vi "Write TIFF Header.vi"(0 "File Path":path, 7 "Image Info":T2, 11 "Error":errorcluster) -> (4 "File Ref":refnum<file>, 8 "Byte Order":T1(ring), 15 "Error":errorcluster)   [LabVIEW 2016]
uses:
  IFD Entry.ctl
  TIF Write Image Information.ctl
panel:
  out "TIF Description":string
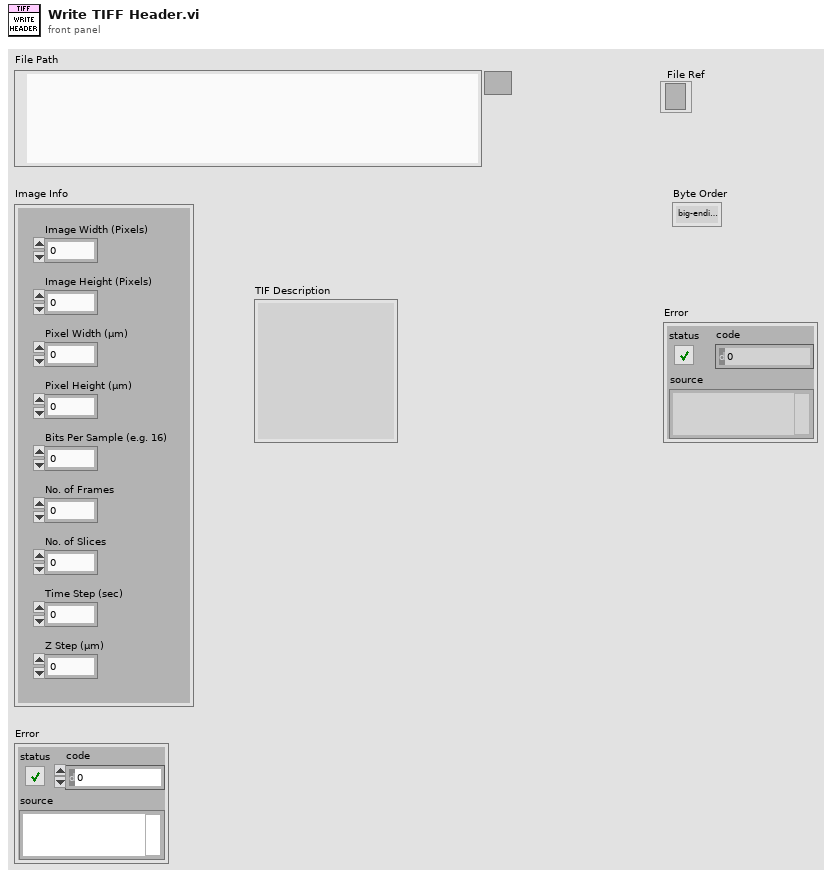
[diagram p1: front panel]
types:
  T1 = enum16{"big-endian, network order", "native, host order", "little-endian"}
  T2 = typedef "TIF Write Image Information.ctl" = cluster{"Image Width (Pixels)":u32, "Image Height (Pixels)":u32, "Pixel Width (µm)":dbl, "Pixel Height (µm)":dbl, "Bits Per Sample (e.g. 16)":u32, "No. of Frames":u32, "No. of Slices":u32, "Time Step (sec)":dbl, "Z Step (µm)":dbl}
  T3 = typedef "IFD Entry.ctl" = cluster{"TIF Tag (U16)":u16, "Data Type (U16)":u16, "Count (U32)":u32, "Value or Offset (U32)":u32, "Write Offset (I64)":i64}
  T4 = enum16{"open", "replace", "create", "open or create", "replace or create", "replace or create with confirmation"}
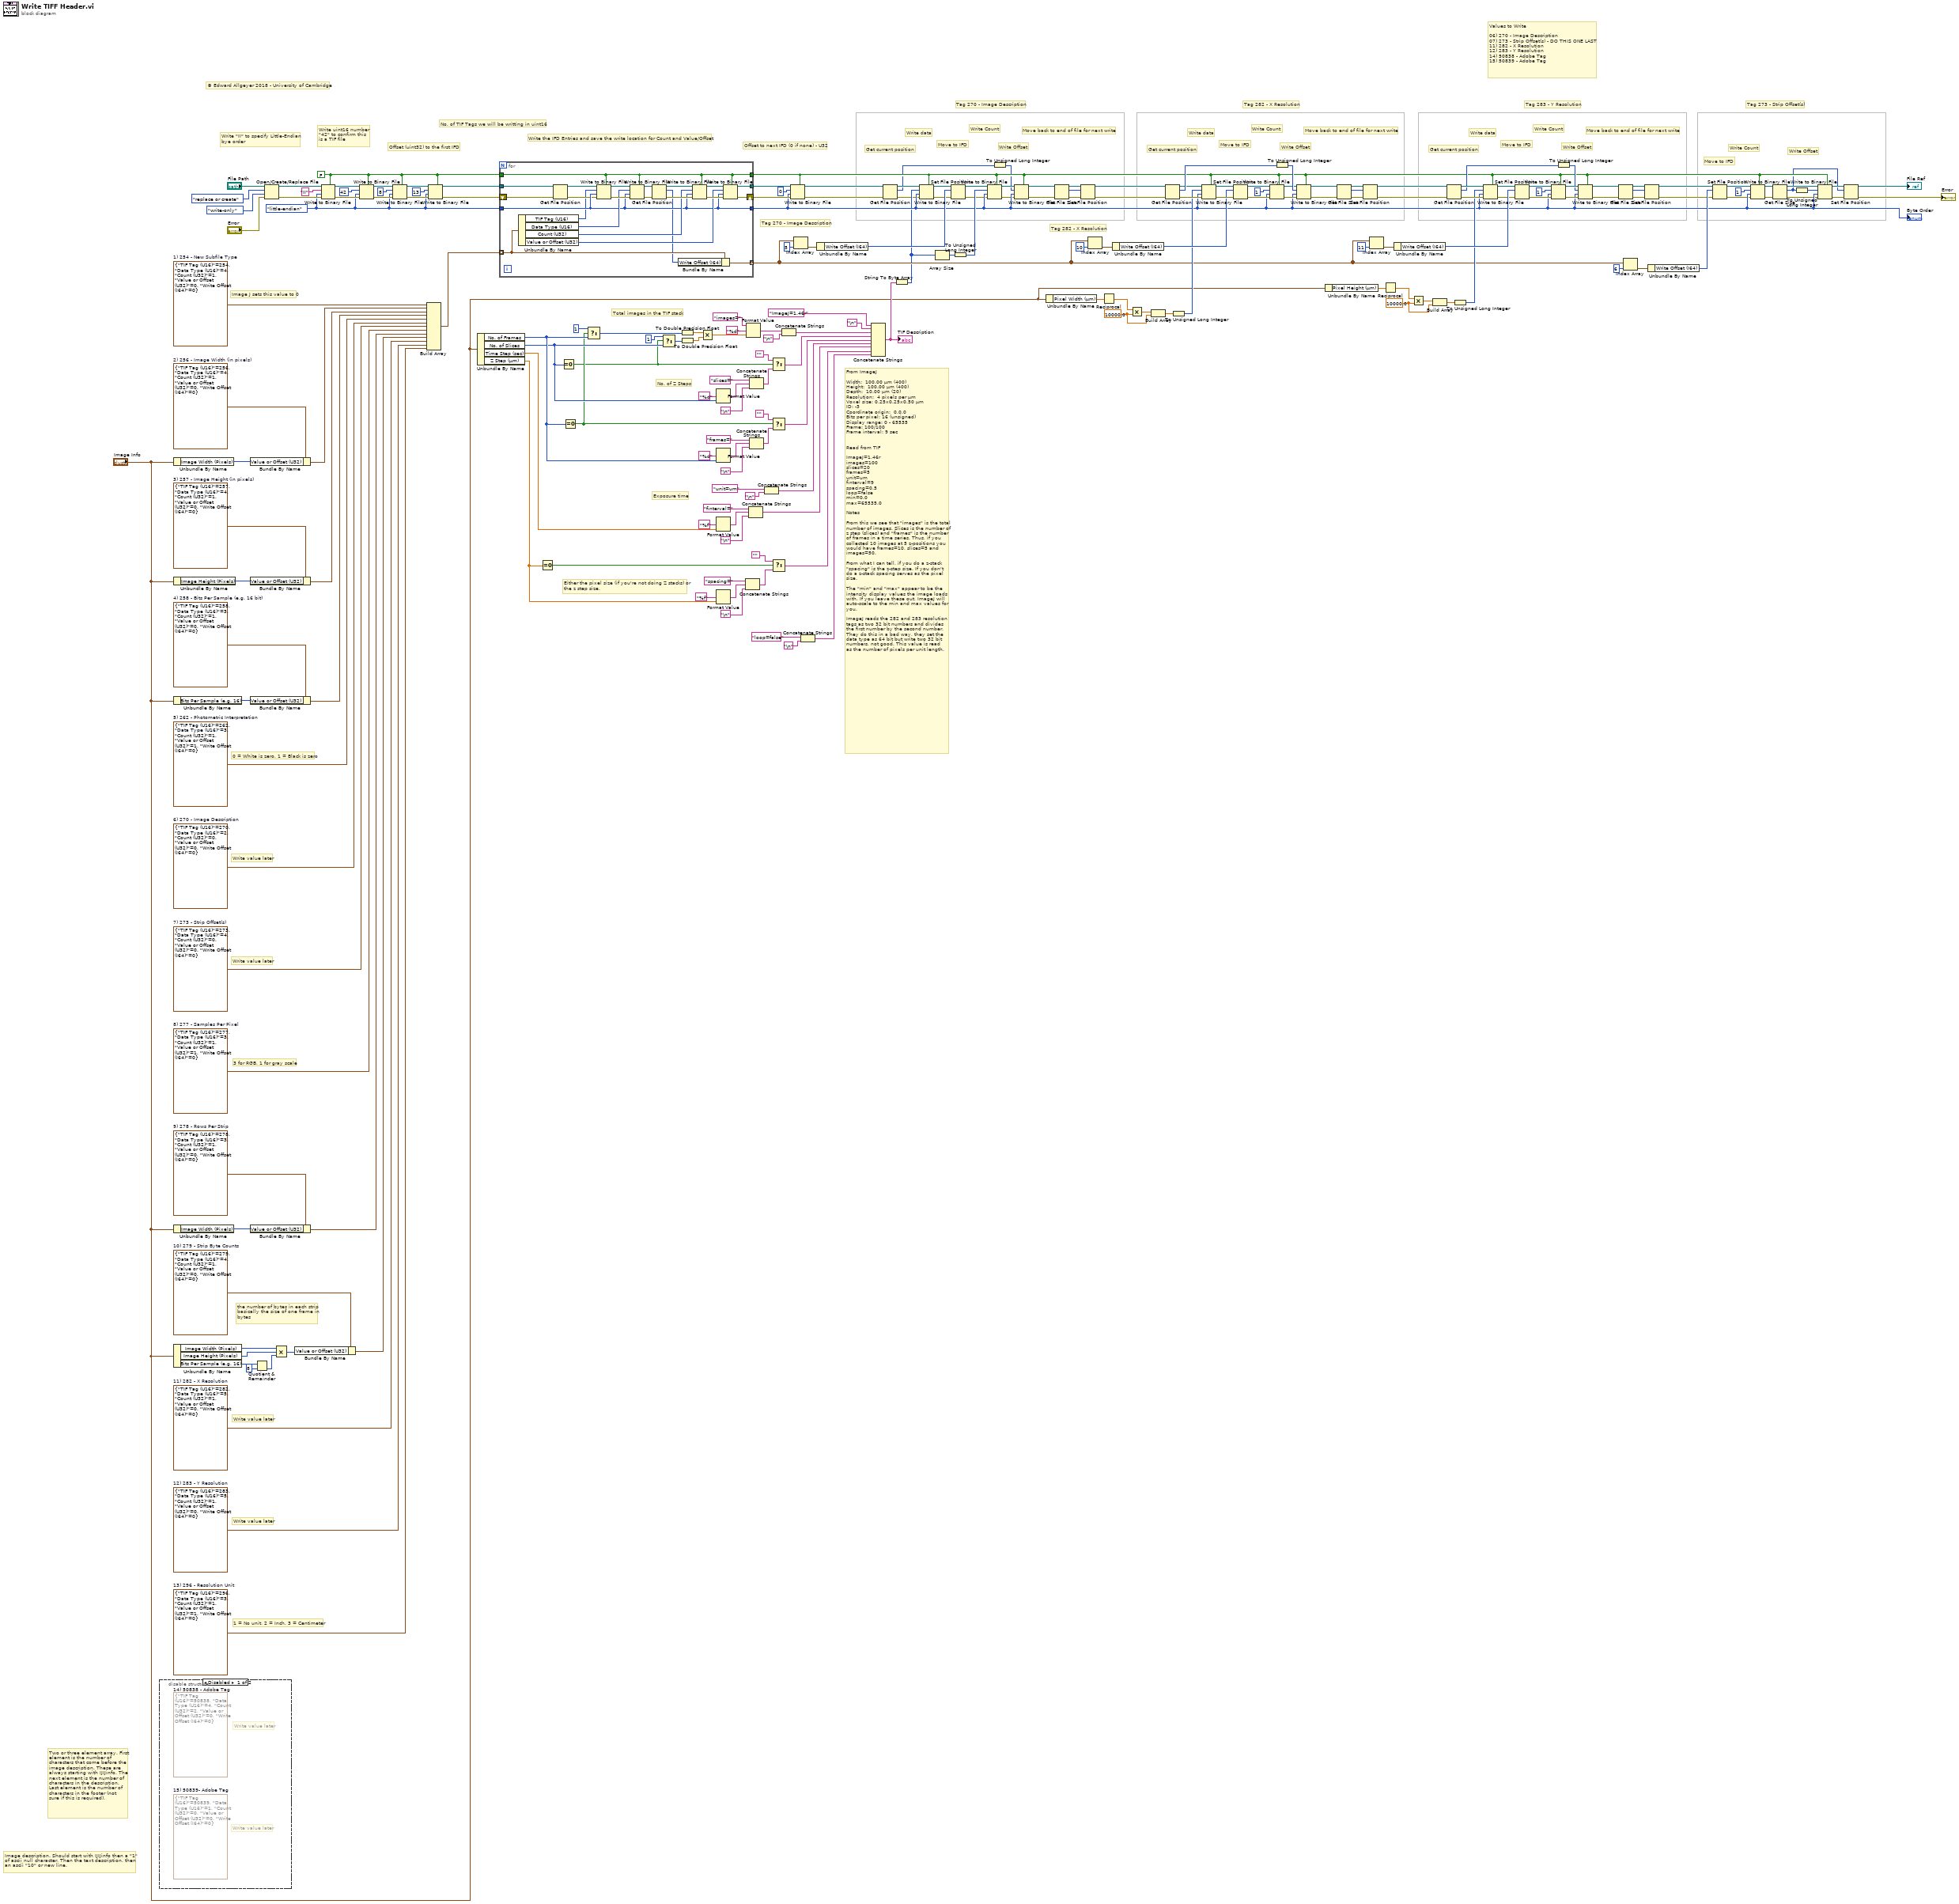
[diagram p0: block diagram]
diagram:
  w82 = 10000.0 ("y")
  w86 = 10000.0 ("y")
  w163 = T3 {"TIF Tag (U16)"=296, "Data Type (U16)"=3, "Count (U32)"=1, "Value or Offset (U32)"=1, "Write Offset (I64)"=0}  # 13) 296 - Resolution Unit
  w164 = T3 {"TIF Tag (U16)"=283, "Data Type (U16)"=5, "Count (U32)"=1, "Value or Offset (U32)"=0, "Write Offset (I64)"=0}  # 12) 283 - Y Resolution
  w165 = T3 {"TIF Tag (U16)"=282, "Data Type (U16)"=5, "Count (U32)"=1, "Value or Offset (U32)"=0, "Write Offset (I64)"=0}  # 11) 282 - X Resolution
  w168 = T3 {"TIF Tag (U16)"=279, "Data Type (U16)"=4, "Count (U32)"=1, "Value or Offset (U32)"=0, "Write Offset (I64)"=0}  # 10) 279 - Strip Byte Counts
  w176 = T3 {"TIF Tag (U16)"=278, "Data Type (U16)"=3, "Count (U32)"=1, "Value or Offset (U32)"=0, "Write Offset (I64)"=0}  # 9) 278 - Rows Per Strip
  w177 = T3 {"TIF Tag (U16)"=277, "Data Type (U16)"=3, "Count (U32)"=1, "Value or Offset (U32)"=1, "Write Offset (I64)"=0}  # 8) 277 - Samples Per Pixel
  w178 = T3 {"TIF Tag (U16)"=273, "Data Type (U16)"=4, "Count (U32)"=0, "Value or Offset (U32)"=0, "Write Offset (I64)"=0}  # 7) 273 - Strip Offset(s)
  w179 = T3 {"TIF Tag (U16)"=270, "Data Type (U16)"=2, "Count (U32)"=0, "Value or Offset (U32)"=0, "Write Offset (I64)"=0}  # 6) 270 - Image Description
  w180 = T3 {"TIF Tag (U16)"=262, "Data Type (U16)"=3, "Count (U32)"=1, "Value or Offset (U32)"=1, "Write Offset (I64)"=0}  # 5) 262 - Photometric Interpretation
  w183 = T3 {"TIF Tag (U16)"=258, "Data Type (U16)"=3, "Count (U32)"=1, "Value or Offset (U32)"=0, "Write Offset (I64)"=0}  # 4) 258 - Bits Per Sample (e.g. 16 bit)
  w186 = T3 {"TIF Tag (U16)"=257, "Data Type (U16)"=4, "Count (U32)"=1, "Value or Offset (U32)"=0, "Write Offset (I64)"=0}  # 3) 257 - Image Height (in pixels)
  w190 = T3 {"TIF Tag (U16)"=256, "Data Type (U16)"=4, "Count (U32)"=1, "Value or Offset (U32)"=0, "Write Offset (I64)"=0}  # 2) 256 - Image Width (in pixels)
  w188 = T3 {"TIF Tag (U16)"=254, "Data Type (U16)"=4, "Count (U32)"=1, "Value or Offset (U32)"=0, "Write Offset (I64)"=0}  # 1) 254 - New Subfile Type
  w158 = FALSE ("prepend array or string size? (T)")
  w159 = T1."little-endian" ("byte order (0:big-endian, network order)")
  # "© Edward Allgeyer 2018 - University of Cambridge"
  # "No. of Z Steps"
  # "Either the pixel size (if you're not doing Z stacks) or\nthe z step size."
  # "Total images in the TIF stack"
  # "Exposure time"
  # "Tag 270 - Image Description"
  # "Move back to end of file for next write"
  # "Move to IFD"
  # "Write data"
  # "Get current position"
  # "Write Offset"
  # "Write Count"
  # "Tag 273 - Strip Offset(s)"
  # "Move to IFD"
  # "Write Offset"
  # "Write Count"
  # "Tag 283 - Y Resolution"
  # "Move back to end of file for next write"
  # "Move to IFD"
  # "Write data"
  # "Get current position"
  # "Write Offset"
  # "Write Count"
  # "Tag 282 - X Resolution"
  # "Tag 282 - X Resolution"
  # "Move back to end of file for next write"
  # "Move to IFD"
  # "Write data"
  # "Get current position"
  # "Write Offset"
  # "Write Count"
  # "Offset to next IFD (0 if none) - U32"
  # "Tag 270 - Image Description"
  # "From ImageJ\n\nWidth:  100.00 µm (400)\nHeight:  100.00 µm (400)\nDepth:  10.00 µm (20)\nResolution:  4 pixels per µm\nVoxel size: 0.25x0.25x0.50 µm\nID: -3\nCoordinate origin:  0,0,0\nBits per pixel: 16 (unsigned)\nDisplay range: 0 - 65535\nFrame: 100/100\nFrame interval: 9 sec\n\n\nRead from TIF\n\nImageJ=1.46r\nimages=100\nslices=20\nframes=5\nunit=um\nfinterval=9\nspacing=0.5\nloop=false\nmin=0.0\nmax=65535.0\n\nNotes\n\nFrom this we see that \"images\" is the total\nnumber of images. Slices is the number of\nz step (slices) and \"frames\" is the number\nof frames in a time series. Thus, if you\ncollected 10 images at 5 z-positions you\nwould have frames=10, slices=5 and\nimages=50.\n\nFrom what I can tell, if you do a z-stack\n\"spacing\" is the z-step size. If you don't\ndo a z-stack spacing serves as the pixel\nsize.\n\nThe \"min\" and \"max\" appear to be the\nintensity display values the image loads\nwith. If you leave these out, ImageJ will\nauto-scale to the min and max values for\nyou.\n\nImageJ reads the 282 and 283 resolution\ntags as two 32 bit numbers and divides\nthe first number by the second number.\nThey do this in a bad way, they set the\ndata type as 64 bit but write two 32 bit\nnumbers, not good. This value is read\nas the number of pixels per unit length."
  # "Values to Write\n\n06) 270 - Image Description\n07) 273 - Strip Offset(s) - DO THIS ONE LAST\n11) 282 - X Resolution\n12) 283 - Y Resolution\n14) 50838 - Adobe Tag\n15) 50839 - Adobe Tag"
  # "Write the IFD Entries and save the write location for Count and Value/Offset"
  # "Image description. Should start with IJIJinfo then a \"1\"\nof ascii null character. Then the text description, then\nan ascii \"10\" or new line."
  # "Two or three element array. First\nelement is the number of\ncharacters that come before the\nimage description. These are\nalways starting with IJIJinfo. The\nnext element is the number of\ncharacters in the description.\nLast element is the number of\ncharacters in the footer (not\nsure if this is required)."
  # "1 = No unit, 2 = Inch, 3 = Centimeter"
  # "Write value later"
  # "Write value later"
  # "the number of bytes in each strip\nbasically the size of one frame in\nbytes"
  # "3 for RGB, 1 for gray scale"
  # "Write value later"
  # "Write value later"
  # "Image J sets this value to 0"
  # "0 = White is zero, 1 = Black is zero"
  # "No. of TIF Tags we will be writting in uint16"
  # "Offset (uint32) to the first IFD"
  # "Write uint16 number\n\"42\" to confirm this\nis a TIF file"
  # "Write \"II\" to specify Little-Endian\nbye order"
  n1 = disable-structure shown="Disabled" {
    frame Disabled {
      (unwired) T3 {"TIF Tag (U16)"=50839, "Data Type (U16)"=1, "Count (U32)"=0, "Value or Offset (U32)"=0, "Write Offset (I64)"=0}  # 15) 50839- Adobe Tag
      (unwired) T3 {"TIF Tag (U16)"=50838, "Data Type (U16)"=4, "Count (U32)"=2, "Value or Offset (U32)"=0, "Write Offset (I64)"=0}  # 14) 50838 - Adobe Tag
      # "Write value later"
      # "Write value later"
    }
    frame Enabled {
    }
  }
  n2 = Unbundle By Name("Image Info") -> ("Image Width (Pixels)"=w189:u32)
  n3 = Unbundle By Name("Image Info") -> ("Image Height (Pixels)"=w185:u32)
  n4 = Unbundle By Name("Image Info") -> ("Bits Per Sample (e.g. 16)"=w182:u32)
  n5 = Unbundle By Name("Image Info") -> ("Image Width (Pixels)"=w175:u32)
  n6 = Unbundle By Name("Image Info") -> ("Image Width (Pixels)"=w171:u32, "Image Height (Pixels)"=w170:u32, "Bits Per Sample (e.g. 16)"=w173:u32)
  n7 = Bundle By Name(cluster=w190, "Value or Offset (U32)"=w189) -> (w187:T3)
  n8 = Bundle By Name(cluster=w186, "Value or Offset (U32)"=w185) -> (w184:T3)
  n9 = Bundle By Name(cluster=w183, "Value or Offset (U32)"=w182) -> (w181:T3)
  n10 = Bundle By Name(cluster=w176, "Value or Offset (U32)"=w175) -> (w174:T3)
  n11 = Quotient & Remainder(x=w173, y=u32 8) -> (floor(x/y)=w169:u32)  [unwired: 1 out]
  n12 = Open/Create/Replace File(file path (use dialog)="File Path", error in="Error", operation (0:open)=T4."replace or create", access (0:read/write)=enum16{"read/write", "read-only", "write-only"}."write-only") -> (refnum out=w2:refnum<file>, error out=w201:errorcluster)  [unwired: 2 in, 1 out]
  n13 = Compound Arithmetic op=MULTIPLY(w171, w170, w169) -> (w167:u32)
  n14 = Bundle By Name(cluster=w168, "Value or Offset (U32)"=w167) -> (w166:T3)
  n15 = Write to Binary File(file (use dialog)=w2, data="II", error in=w201, 5:w158, 9:w159) -> (refnum out=w196:refnum<file>, error out=w200:errorcluster)  [unwired: 1 in, 1 out]
  n16 = Write to Binary File(file (use dialog)=w196, data=u16 42, error in=w200, 5:w158, 9:w159) -> (refnum out=w195:refnum<file>, error out=w198:errorcluster)  [unwired: 1 in, 1 out]
  n17 = Write to Binary File(file (use dialog)=w195, data=u32 8, error in=w198, 5:w158, 9:w159) -> (refnum out=w194:refnum<file>, error out=w193:errorcluster)  [unwired: 1 in, 1 out]
  n18 = Build Array(w188, w187, w184, w181, w180, w179, w178, w177, w174, w166, w165, w164, w163) -> (w160:T3[])
  n19 = Write to Binary File(file (use dialog)=w194, data=u16 13, error in=w193, 5:w158, 9:w159) -> (refnum out=w162:refnum<file>, error out=w161:errorcluster)  [unwired: 1 in, 1 out]
  n20 = Unbundle By Name("Image Info") -> ("No. of Frames"=w138:u32, "No. of Slices"=w135:u32, "Time Step (sec)"=w144:dbl, "Z Step (µm)"=w127:dbl)
  n21 = for {
    tunnel: w162 -> [w210]
    tunnel: w160 -> [w216] mode=indexing
    tunnel: w158 -> [w212]
    shift-right: [w217] -> w116
    shift-left: w161 -> [w208]
    tunnel: [w215] -> w55 mode=indexing
    tunnel: [w214] -> w117
    tunnel: w159 -> [w213]
    tunnel: [w213] -> w51
    tunnel: [w212] -> w52
    n22 = Unbundle By Name(w216) -> ("TIF Tag (U16)"=w206:u16, "Data Type (U16)"=w226:u16, "Count (U32)"=w221:u32, "Value or Offset (U32)"=w218:u32)
    n23 = Get File Position(4:w208, 7:w210) -> (0:w207:errorcluster, 3:w209:refnum<file>)  [unwired: 1 out]
    n24 = Write to Binary File(file (use dialog)=w209, data=w206, error in=w207, 5:w212, 9:w213) -> (refnum out=w228:refnum<file>, error out=w227:errorcluster)  [unwired: 1 in, 1 out]
    n25 = Write to Binary File(file (use dialog)=w228, data=w226, error in=w227, 5:w212, 9:w213) -> (refnum out=w225:refnum<file>, error out=w224:errorcluster)  [unwired: 1 in, 1 out]
    n26 = Get File Position(4:w224, 7:w225) -> (0:w222:errorcluster, 2:w211:i64, 3:w223:refnum<file>)
    n27 = Bundle By Name(cluster=w216, "Write Offset (I64)"=w211) -> (w215:T3)
    n28 = Write to Binary File(file (use dialog)=w223, data=w221, error in=w222, 5:w212, 9:w213) -> (refnum out=w220:refnum<file>, error out=w219:errorcluster)  [unwired: 1 in, 1 out]
    n29 = Write to Binary File(file (use dialog)=w220, data=w218, error in=w219, 5:w212, 9:w213) -> (refnum out=w214:refnum<file>, error out=w217:errorcluster)  [unwired: 1 in, 1 out]
  }
  "Byte Order" <- w51
  n30 = Equal To 0?(x=w127) -> (x = 0?=w128:bool)
  n31 = Equal To 0?(x=w135) -> (x = 0?=w119:bool)
  n32 = Equal To 0?(x=w138) -> (x = 0?=w120:bool)
  n33 = Select(t=u32 1, s=w120, f=w138) -> (s? t:f=w134:u32)
  n34 = Select(t=u32 1, s=w119, f=w135) -> (s? t:f=w133:u32)
  n35 = To Double Precision Float(number=w134) -> (double precision float=w157:dbl)
  n36 = To Double Precision Float(number=w133) -> (double precision float=w156:dbl)
  n37 = Multiply(x=w157, y=w156) -> (x*y=w155:dbl)
  n38 = Format Value(format string="%d", value (0)=w135) -> (output string=w149:string)  [unwired: 1 in]
  n39 = Format Value(format string="%d", value (0)=w138) -> (output string=w141:string)  [unwired: 1 in]
  n40 = Format Value(format string="%f", value (0)=w144) -> (output string=w151:string)  [unwired: 1 in]
  n41 = Format Value(format string="%f", value (0)=w127) -> (output string=w131:string)  [unwired: 1 in]
  n42 = Concatenate Strings("spacing=", w131, "\n") -> (w132:string)
  n43 = Format Value(string ("")="images=", format string="%d", value (0)=w155) -> (output string=w125:string)
  n44 = Concatenate Strings("finterval=", w151, "\n") -> (w53:string)
  n45 = Concatenate Strings("slices=", w149, "\n") -> (w150:string)
  n46 = Concatenate Strings("frames=", w141, "\n") -> (w140:string)
  n47 = Concatenate Strings("unit=um", "\n") -> (w14:string)
  n48 = Select(t="", s=w119, f=w150) -> (s? t:f=w123:string)
  n49 = Select(t="", s=w120, f=w140) -> (s? t:f=w122:string)
  n50 = Select(t="", s=w128, f=w132) -> (s? t:f=w121:string)
  n51 = Concatenate Strings(w125, "\n") -> (w124:string)
  n52 = Write to Binary File(file (use dialog)=w117, data=u32 0, error in=w116, 5:w52, 9:w51) -> (refnum out=w113:refnum<file>, error out=w112:errorcluster)  [unwired: 1 in, 1 out]
  n53 = Index Array(array=w55, index=5) -> (element=w114:T3)
  n54 = Concatenate Strings("loop=false", "\n") -> (w11:string)
  n55 = Unbundle By Name(w114) -> ("Write Offset (I64)"=w111:i64)
  n56 = Concatenate Strings("ImageJ=1.46r", "\n", w124, w123, w122, w14, w53, w121, w11) -> (w10:string)
  "TIF Description" <- w10
  n57 = Get File Position(4:w112, 7:w113) -> (0:w34:errorcluster, 2:w29:i64, 3:w35:refnum<file>)
  n58 = String To Byte Array(string=w10) -> (unsigned byte array=w36:u8[])
  n59 = Write to Binary File(file (use dialog)=w35, data=w36, error in=w34, 5:w52, 9:w51) -> (refnum out=w22:refnum<file>, error out=w21:errorcluster)  [unwired: 1 in, 1 out]
  n60 = Array Size(array=w36) -> (size(s)=w37:i32)
  n61 = Set File Position(offset (in bytes) (0)=w111, refnum=w22, error in=w21) -> (refnum out=w33:refnum<file>, error out=w32:errorcluster)  [unwired: 1 in]
  n62 = To Unsigned Long Integer(number=w37) -> (unsigned 32bit integer=w110:u32)
  n63 = Write to Binary File(file (use dialog)=w33, data=w110, error in=w32, 5:w52, 9:w51) -> (refnum out=w31:refnum<file>, error out=w30:errorcluster)  [unwired: 1 in, 1 out]
  n64 = To Unsigned Long Integer(number=w29) -> (unsigned 32bit integer=w28:u32)
  n65 = Write to Binary File(file (use dialog)=w31, data=w28, error in=w30, 5:w52, 9:w51) -> (refnum out=w27:refnum<file>, error out=w24:errorcluster)  [unwired: 1 in, 1 out]
  n66 = Unbundle By Name("Image Info") -> ("Pixel Width (µm)"=w88:dbl)
  n67 = Get File Size(file=w27, error in=w24) -> (refnum out=w26:refnum<file>, size (in bytes)=w25:i64, 0:w23:errorcluster)
  n68 = Set File Position(offset (in bytes) (0)=w25, refnum=w26, error in=w23) -> (refnum out=w93:refnum<file>, error out=w92:errorcluster)  [unwired: 1 in]
  n69 = Index Array(array=w55, index=10) -> (element=w91:T3)
  n70 = Reciprocal(x=w88) -> (1/x=w4:dbl)
  n71 = Unbundle By Name(w91) -> ("Write Offset (I64)"=w90:i64)
  n72 = Multiply(x=w4, y=w86) -> (x*y=w87:dbl)
  n73 = Build Array(w87, w86) -> (w85:dbl[])
  n74 = Get File Position(4:w92, 7:w93) -> (0:w95:errorcluster, 2:w100:i64, 3:w94:refnum<file>)
  n75 = To Unsigned Long Integer(number=w85) -> (unsigned 32bit integer=w84:u32[])
  n76 = Write to Binary File(file (use dialog)=w94, data=w84, error in=w95, 5:w52, 9:w51) -> (refnum out=w107:refnum<file>, error out=w108:errorcluster)  [unwired: 1 in, 1 out]
  n77 = Set File Position(offset (in bytes) (0)=w90, refnum=w107, error in=w108) -> (refnum out=w96:refnum<file>, error out=w97:errorcluster)  [unwired: 1 in]
  n78 = Write to Binary File(file (use dialog)=w96, data=u32 1, error in=w97, 5:w52, 9:w51) -> (refnum out=w98:refnum<file>, error out=w99:errorcluster)  [unwired: 1 in, 1 out]
  n79 = To Unsigned Long Integer(number=w100) -> (unsigned 32bit integer=w101:u32)
  n80 = Write to Binary File(file (use dialog)=w98, data=w101, error in=w99, 5:w52, 9:w51) -> (refnum out=w102:refnum<file>, error out=w105:errorcluster)  [unwired: 1 in, 1 out]
  n81 = Unbundle By Name("Image Info") -> ("Pixel Height (µm)"=w80:dbl)
  n82 = Get File Size(file=w102, error in=w105) -> (refnum out=w103:refnum<file>, size (in bytes)=w104:i64, 0:w106:errorcluster)
  n83 = Set File Position(offset (in bytes) (0)=w104, refnum=w103, error in=w106) -> (refnum out=w60:refnum<file>, error out=w59:errorcluster)  [unwired: 1 in]
  n84 = Index Array(array=w55, index=11) -> (element=w77:T3)
  n85 = Reciprocal(x=w80) -> (1/x=w6:dbl)
  n86 = Unbundle By Name(w77) -> ("Write Offset (I64)"=w78:i64)
  n87 = Multiply(x=w6, y=w82) -> (x*y=w81:dbl)
  n88 = Build Array(w81, w82) -> (w83:dbl[])
  n89 = Get File Position(4:w59, 7:w60) -> (0:w75:errorcluster, 2:w70:i64, 3:w76:refnum<file>)
  n90 = To Unsigned Long Integer(number=w83) -> (unsigned 32bit integer=w58:u32[])
  n91 = Write to Binary File(file (use dialog)=w76, data=w58, error in=w75, 5:w52, 9:w51) -> (refnum out=w63:refnum<file>, error out=w62:errorcluster)  [unwired: 1 in, 1 out]
  n92 = Set File Position(offset (in bytes) (0)=w78, refnum=w63, error in=w62) -> (refnum out=w74:refnum<file>, error out=w73:errorcluster)  [unwired: 1 in]
  n93 = Write to Binary File(file (use dialog)=w74, data=u32 1, error in=w73, 5:w52, 9:w51) -> (refnum out=w72:refnum<file>, error out=w71:errorcluster)  [unwired: 1 in, 1 out]
  n94 = To Unsigned Long Integer(number=w70) -> (unsigned 32bit integer=w69:u32)
  n95 = Write to Binary File(file (use dialog)=w72, data=w69, error in=w71, 5:w52, 9:w51) -> (refnum out=w68:refnum<file>, error out=w65:errorcluster)  [unwired: 1 in, 1 out]
  n96 = Get File Size(file=w68, error in=w65) -> (refnum out=w67:refnum<file>, size (in bytes)=w66:i64, 0:w64:errorcluster)
  n97 = Index Array(array=w55, index=6) -> (element=w56:T3)
  n98 = Set File Position(offset (in bytes) (0)=w66, refnum=w67, error in=w64) -> (refnum out=w47:refnum<file>, error out=w46:errorcluster)  [unwired: 1 in]
  n99 = Unbundle By Name(w56) -> ("Write Offset (I64)"=w54:i64)
  n100 = Set File Position(offset (in bytes) (0)=w54, refnum=w47, error in=w46) -> (refnum out=w49:refnum<file>, error out=w50:errorcluster)  [unwired: 1 in]
  n101 = Write to Binary File(file (use dialog)=w49, data=u32 1, error in=w50, 5:w52, 9:w51) -> (refnum out=w45:refnum<file>, error out=w44:errorcluster)  [unwired: 1 in, 1 out]
  n102 = Get File Size(file=w45, error in=w44) -> (refnum out=w42:refnum<file>, size (in bytes)=w38:i64, 0:w43:errorcluster)
  n103 = To Unsigned Long Integer(number=w38) -> (unsigned 32bit integer=w41:u32)
  n104 = Write to Binary File(file (use dialog)=w42, data=w41, error in=w43, 5:w52, 9:w51) -> (refnum out=w40:refnum<file>, error out=w39:errorcluster)  [unwired: 1 in, 1 out]
  n105 = Set File Position(offset (in bytes) (0)=w38, refnum=w40, error in=w39) -> (refnum out=→"File Ref":refnum<file>, error out=→"Error":errorcluster)  [unwired: 1 in]
